vi "2layer_Neuron.vi"(1 "Offset":dbl, 2 "Weights_2layer":fxp<+/-,32,8>[](array[numeric]), 3 "Array_Out_hx":fxp<+/-,32,8>[](array[numeric])) -> (0 "Output":fxp<+/-,32,8>)   [LabVIEW 2016]
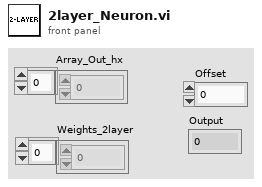
[diagram p1: front panel]
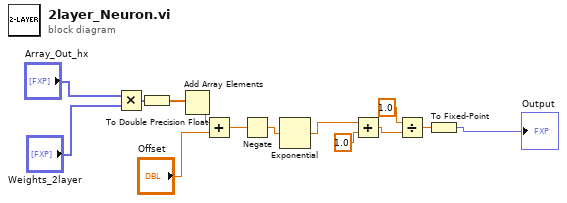
[diagram p0: block diagram]
diagram:
  n1 = Multiply(x="Array_Out_hx", y="Weights_2layer") -> (x*y=w4:fxp<+/-,64,16>[])
  n2 = To Double Precision Float(number=w4) -> (double precision float=w3:dbl[])
  n3 = Add Array Elements(numeric array=w3) -> (sum=w7:dbl)
  n4 = Add(x=w7, y="Offset") -> (x+y=w5:dbl)
  n5 = Negate(x=w5) -> (-x=w11:dbl)
  n6 = Exponential(1:w11) -> (0:w10:dbl)
  n7 = Add(x=w10, y=1.0) -> (x+y=w13:dbl)
  n8 = Divide(x=1.0, y=w13) -> (x/y=w2:dbl)
  n9 = To Fixed-Point(number=w2) -> (fixed-point=→"Output":fxp<+/-,32,8>)  [unwired: 1 in]
